vi "Update-temperature-graph-axes.vi"(8 "error in (no error)":errorcluster, 9 "Temperature graph":refnum<vi>, 10 "Config params in":refnum<data-value>, 11 "Temperature params in":refnum<data-value>) -> (0 "error out":errorcluster)   [LabVIEW 2013, in "CameraVision.lvlib" / "CV-Temperature.lvclass"]
uses:
  CV-Temperature.lvclass
  Configuration/CV-Configuration.lvclass
  Configuration/CV-Configuration.lvclass/CV-Configuration.ctl
  CV-Temperature.lvclass/CV-Temperature.ctl
  Read Axis origin relative position.vi
  Configuration/Read ROI width.vi
  Configuration/Read ROI height.vi
  Configuration/Read Width scale.vi
  Configuration/Read Height scale.vi
  Write X-scale.vi
  Write Y-scale.vi
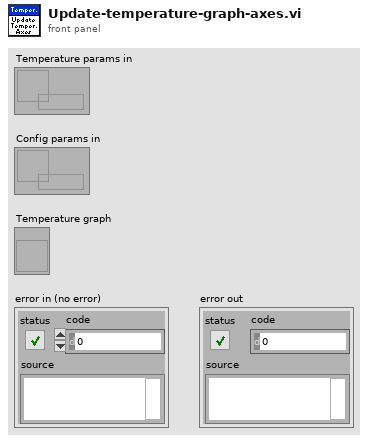
[diagram p1: front panel]
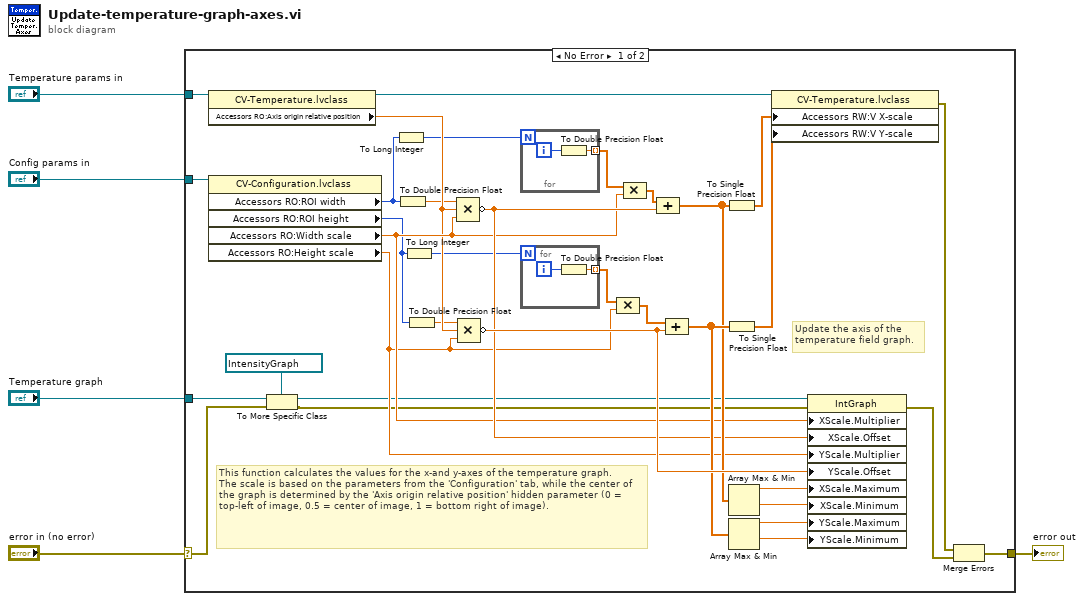
[diagram p0: block diagram]
diagram:
  n1 = case shown="No Error" "error in (no error)" {
    selector: "error in (no error)" -> [w7 w44]
    tunnel: "Temperature graph" -> [w10 _]
    tunnel: "Config params in" -> [w39 _]
    tunnel: "Temperature params in" -> [w38 _]
    tunnel: [w18 w44] -> w2
    frame No Error {
      # "This function calculates the values for the x-and y-axes of the temperature graph.\nThe scale is based on the parameters from the 'Configuration' tab, while the center of the graph is determined by the 'Axis origin relative position' hidden parameter (0 = top-left of image, 0.5 = center of image, 1 = bottom right of image)."
      # "Update the axis of the \ntemperature field graph."
      n2 = property class="CV-Temperature.lvclass"(reference=w38) -> (reference out=w34:refnum<data-value>, "Accessors RO:Axis origin relative position"=w15:dbl)  [unwired: 1 in, 1 out]
      n3 = property class="CV-Configuration.lvclass"(reference=w39) -> ("Accessors RO:ROI width"=w16:u32, "Accessors RO:ROI height"=w17:u32, "Accessors RO:Width scale"=w25:dbl, "Accessors RO:Height scale"=w24:dbl)  [unwired: 1 in, 2 out]
      n4 = To More Specific Class(target class=refnum<vi> refnum ("Temperature graph"), reference=w10, error in=w7) -> (specific class reference=w9:refnum<vi>, error out=w6:errorcluster)
      n5 = To Long Integer(number=w16) -> (32bit integer=w14:i32)
      n6 = To Double Precision Float(number=w16) -> (double precision float=w11:dbl)
      n7 = To Long Integer(number=w17) -> (32bit integer=w13:i32)
      n8 = To Double Precision Float(number=w17) -> (double precision float=w12:dbl)
      n9 = Compound Arithmetic op=MULTIPLY(w11, w15, w25) -> (invert w26:dbl)
      n10 = Compound Arithmetic op=MULTIPLY(w12, w15, w24) -> (invert w33:dbl)
      n11 = for {
        N: w14 -> [_]
        tunnel: [w40] -> w19 mode=indexing
        i -> [w41]
        n12 = To Double Precision Float(number=w41) -> (double precision float=w40:dbl)
      }
      n13 = for {
        N: w13 -> [_]
        tunnel: [w42] -> w21 mode=indexing
        i -> [w43]
        n14 = To Double Precision Float(number=w43) -> (double precision float=w42:dbl)
      }
      n15 = Compound Arithmetic op=MULTIPLY(w21, w24) -> (w22:dbl[])
      n16 = Compound Arithmetic op=MULTIPLY(w19, w25) -> (w20:dbl[])
      n17 = Compound Arithmetic op=ADD(w20, w26) -> (w29:dbl[])
      n18 = Compound Arithmetic op=ADD(w22, w33) -> (w32:dbl[])
      n19 = To Single Precision Float(number=w29) -> (single precision float=w35:sgl[])
      n20 = To Single Precision Float(number=w32) -> (single precision float=w36:sgl[])
      n21 = Array Max & Min(array=w29) -> (max value=w27:dbl, min value=w28:dbl)  [unwired: 2 out]
      n22 = Array Max & Min(array=w32) -> (max value=w30:dbl, min value=w31:dbl)  [unwired: 2 out]
      n23 = property class="CV-Temperature.lvclass"(reference=w34, "Accessors RW:V X-scale"=w35, "Accessors RW:V Y-scale"=w36) -> (error out=w37:errorcluster)  [unwired: 1 in, 1 out]
      n24 = property class="IntGraph"(reference=w9, error in=w6, "XScale.Multiplier"=w25, "XScale.Offset"=w26, "YScale.Multiplier"=w24, "YScale.Offset"=w33, "XScale.Maximum"=w27, "XScale.Minimum"=w28, "YScale.Maximum"=w30, "YScale.Minimum"=w31) -> (error out=w23:errorcluster)  [unwired: 1 out]
      n25 = Merge Errors(w37, w23) -> (w18:errorcluster)
    }
    frame Error {
    }
  }
  "error out" <- w2
